vi "Read Exception Status.vi"(8 "error in":errorcluster, 11 "Modbus instance in":refnum<class "Modbus API.lvclass">) -> (0 "error out":errorcluster, 2 "exception status":u8, 3 "Modbus instance out":refnum<class "Modbus API.lvclass">)   [LabVIEW 2014, in "MyLib.lvlib" / "Modbus API.lvclass"]
doc: "Interface to reads any exception status set in the device. The exeption status is a set of 8 status bits, packed as a U8 integer. With third-party devices, this function should only be used if the device is a serial device, as the Modbus specification defines this as a serial-only function. However, this library includes support for this function regardless of the transport mechanism."
uses:
  Modbus API.lvclass
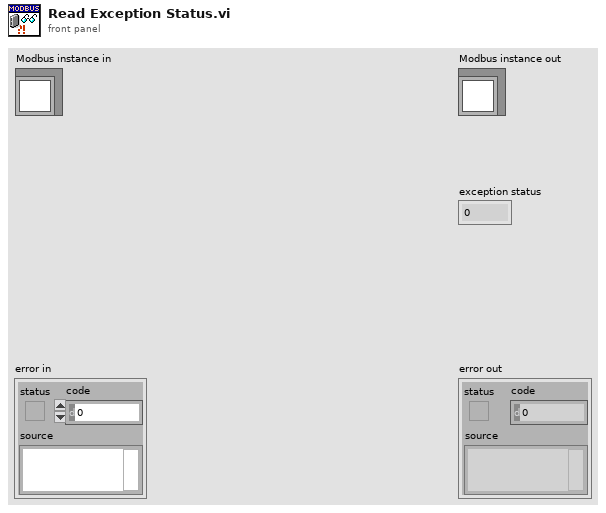
[diagram p1: front panel]
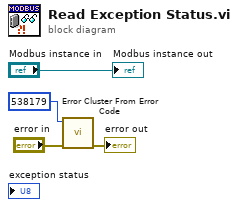
[diagram p0: block diagram]
diagram:
  n1 = call <vilib>:"Error Cluster From Error Code.vi"("error in (no error)"="error in", "error code (0)"=538179) -> ("error out"=→"error out":errorcluster)  [unwired: 7 in]
  "Modbus instance out" <- "Modbus instance in"
